vi "New.vi"(11 "VISA resource name":refnum<visa-resource-name>) -> (0 "error out":errorcluster, 3 "AlphaStep One out":refnum<class "AlphaStep One.lvclass">)   [LabVIEW 2015, in "AlphaStep One.lvclass"]
uses:
  AlphaStep One.lvclass
  AlphaStep One.lvclass/AlphaStep One.ctl
  Serial Device/Serial Device.lvclass
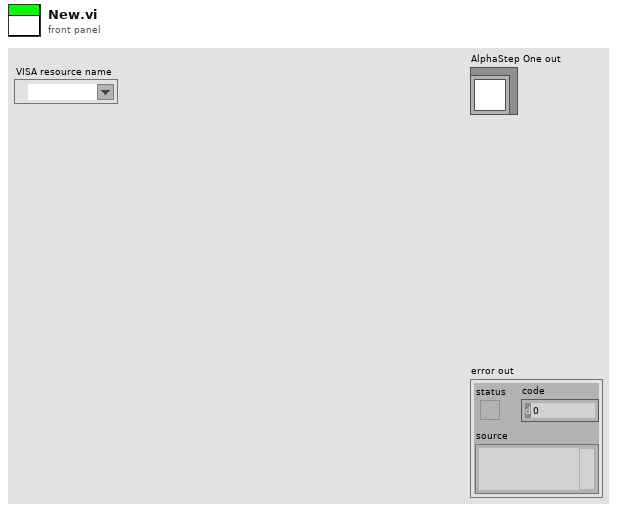
[diagram p1: front panel]
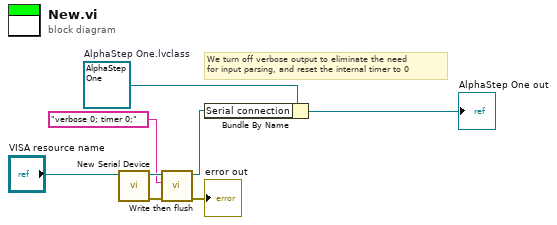
[diagram p0: block diagram]
diagram:
  w7 = refnum<class "AlphaStep One.lvclass"> refnum  # AlphaStep One.lvclass
  # "We turn off verbose output to eliminate the need\nfor input parsing, and reset the internal timer to 0"
  n1 = call "New Serial Device.vi"("VISA resource name"="VISA resource name") -> ("error out"=w3:errorcluster, "Serial Device out"=w5:refnum<class "Serial Device.lvclass">)  [unwired: 9 in]
  n2 = call "Write then flush.vi"("error in (no error)"=w3, "TX Data"="verbose 0; timer 0;", "Serial Device in"=w5) -> ("error out"=→"error out":errorcluster, "Serial Device out"=w1:refnum<class "Serial Device.lvclass">)  [unwired: 7 in]
  n3 = Bundle By Name(cluster=w7, "Serial connection"=w1) -> (→"AlphaStep One out":refnum<class "AlphaStep One.lvclass">)
